vi "APRSGetData.vi"(8 "error in (no error)":errorcluster, 11 "conRef":T1) -> (0 "error out":errorcluster, 1 "APRS packet":string, 3 "conRef out":T1)   [LabVIEW 2012]
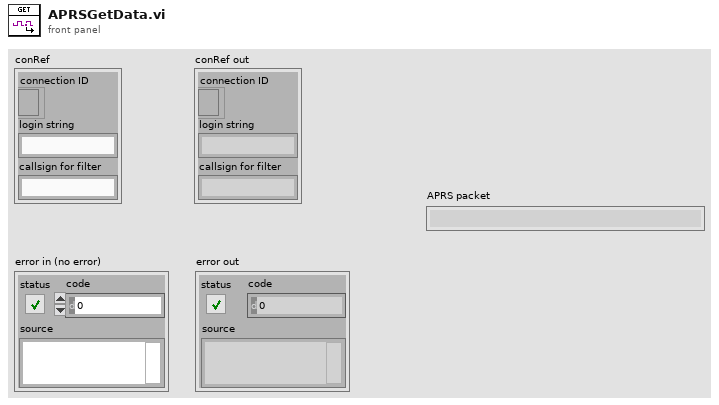
[diagram p1: front panel]
types:
  T1 = cluster{"connection ID":refnum<k5>, "login string":string, "callsign for filter":string}
  T2 = enum16{"Standard", "Buffered", "CRLF", "Immediate"}
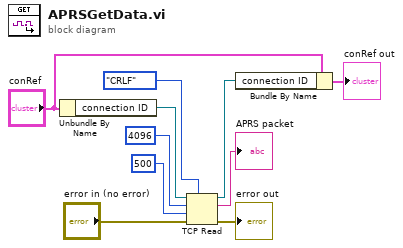
[diagram p0: block diagram]
diagram:
  n1 = Unbundle By Name("conRef") -> ("connection ID"=w6:refnum<k5>)
  n2 = TCP Read(connection ID=w6, bytes to read=4096, error in (no error)="error in (no error)", 7:T2."CRLF" ("mode (standard)"), 9:500 ("timeout ms (25000)")) -> (connection ID out=w4:refnum<k5>, data out=→"APRS packet":string, error out=→"error out":errorcluster)
  n3 = Bundle By Name(cluster="conRef", "connection ID"=w4) -> (→"conRef out":T1)
